vi "Main Page.vi"(8 "error in (no error)":errorcluster, 11 "Node Ptr":T3 format="%.0x") -> (0 "error out":errorcluster)   [LabVIEW 2023, in "Instrument Addon System Explorer.lvlib"]
uses:
  Instrument Addon System Explorer.lvlib
  <vilib>/NI VeriStand/Custom Device API/Custom Device Item Ref.ctl
  Addon Shared/Types/FG Control.ctl
  <vilib>/NI/NI VeriStand Hardware Resource Discovery/_Types/Filter Type.ctl
  Addon Shared/SubVIs/Constants.vi
  <vilib>/NI/NI VeriStand Advanced SysDef API/SysDef API/SysDef.Property.Get.vi
  <vilib>/NI/NI VeriStand Advanced SysDef API/_SubVIs/SysDef.Property.Get.String.vi
  <vilib>/NI/NI VeriStand Advanced SysDef API/SysDef API/SysDef.Property.Set.vi
  <vilib>/NI/NI VeriStand Advanced SysDef API/_SubVIs/SysDef.Property.Set.String.vi
  <vilib>/NI VeriStand/Custom Device API/NI VeriStand - Get Item Property.vi
  <vilib>/NI VeriStand/Custom Device API/Get Item Property (Boolean).vi
  <vilib>/NI VeriStand/Custom Device API/Get Item Property (U32).vi
  <vilib>/NI VeriStand/Custom Device API/Get Item Property (String).vi
  <vilib>/NI VeriStand/Custom Device API/NI VeriStand - Set Item Property.vi
  <vilib>/NI VeriStand/Custom Device API/Set Item Property (Boolean).vi
  <vilib>/NI VeriStand/Custom Device API/Set Item Property (U32).vi
  <vilib>/NI VeriStand/Custom Device API/Set Item Property (String).vi
  <vilib>/Utility/LVClass/Get LV Class Default Value.vi
  Includes/Protocols.lvlibp/Protocol Parent/Protocol Parent.lvclass
  <vilib>/NI VeriStand/Custom Device API/Custom Device API.lvlib
  Addon Shared/Instrument Addon Shared.lvlib
  <vilib>/NI/NI VeriStand Hardware Resource Discovery/NIVS Hardware Discovery.lvlib
  APIs/Scripting API/Instrument Addon Scripting API.lvlib
panel:
  out "Version":string
  in  "PCL Decimation":u32=1 min=1 max=10000 step=1
  in  "Protocol Settings":T1(tab)=enum."TCP/IP"
  in  "4wireMode":bool=TRUE caption="Specify Wire Mode"
  in  "COM Browse":bool
  in  "Termination Character":u8=10 format="%.0x"
  in  "End Write":bool=TRUE caption="End Write on Termination Character?"
  in  "End Read":bool=TRUE caption="End Read on Termination Character?"
  in  "XOFF":T2(ring)=enum."DC3"
  in  "XON":T2(ring)=enum."DC1"
  in  "Flow Control":u16(ring) items=["None"=0, "XON/XOFF"=1, "RTS/CTS"=2, "DTR/DSR"=4]
  in  "Stop Bits":u16(ring)=10 items=["1.0"=10, "1.5"=15, "2.0"=20]
  in  "Parity":enum16{"None", "Odd", "Even", "Mark", "Space"}(ring)
  in  "Data Bits":u16=8 min=5 max=8 step=1
  in  "Baud Rate":u32(ring)=9600 items=["75"=75, "110"=110, "134"=134, "150"=150, "300"=300, "600"=600, "1200"=1200, "1800"=1800, "2400"=2400, "4800"=4800, "7200"=7200, "9600"=9600, "14400"=14400, "19200"=19200, "28800"=28800, "38400"=38400, "56000"=56000, "57600"=57600, "115200"=115200, "128000"=128000, "230400"=230400, "460800"=460800, "921600"=921600, "1843200"=1843200, "3000000"=3000000]
  in  "Port":string="COM1"
  in  "WireMode":i16(ring)=-1 items=["Unknown"=-1, "RS485/Wire4"=0, "RS485/Wire2-EchoDTR"=1, "RS485/Wire2-CtrlDTR"=2, "RS485/Wire2-Auto"=3, "RS232/DTE"=128, "RS232/DCE"=129, "RS232/Auto"=130]
  in  "Assert DTR":bool=TRUE
  in  "VISA Browse":bool
  in  "Append Write Termination Character":bool caption="Append Write Termination Character?"
  in  "Timeout":u32=2000 caption="Timeout (ms)"
  in  "Termination Character":u8=10 format="%.0x"
  in  "Enable Termination Character":bool=TRUE caption="Enable Termination Character?"
  in  "VISA Resource":string="GPIB0::2::INSTR"
  in  "Port":u16
  in  "IP Address":string="localhost"
  in  "UDP Browse":bool
  in  "Target Port":u16
  in  "Target IP Address":string="localhost"
  in  "Local Port":u16
  in  "Local IP Address":string="localhost"
  in  "Assert REN w/ IFC":bool=TRUE caption="Assert REN w/ IFC?"
  in  "IST Bit Sense":bool=TRUE caption="IST Bit Sense?"
  in  "System Controller":bool=TRUE caption="System Controller?"
  in  "GPIB Address":string="1"
  in  "ConvBox Address":string="0"
  in  "ConvBox Browse":bool
  in  "ConvBox Port":string="COM1"
  in  "Protocol":string(combo)
  in  "SHDocVw.IWebBrowser":refnum<k7>(container)
  in  "Header":cluster{"Section Name":string}={"Section Name"="Addon Settings"}
  in  "Description":string
  in  "Name":string
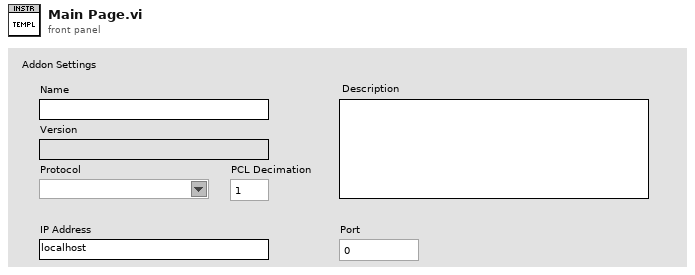
[diagram p1: front panel]
types:
  T1 = enum32{"RS232", "VISA", "TCP/IP", "UDP", "ConvBox"}
  T2 = enum16{"NUL", "SOH", "STX", "ETX", "EOT", "ENQ", "ACK", "BEL", "BS", "HT", "LF", "VT", "FF", "CR", "SO", "SI", "DLE", "DC1", "DC2", "DC3", "DC4", "NAK", "SYN", "ETB", "CAN", "EM", "SUB", "ESC", "FS", "GS", "RS", "US", "SP", "!", "\"", "#", "$", "%", "&", "'", "(", ")", "*", "+", ",", "- (-)", ".", "/", "0", "1", "2", "3", "4", "5", "6", "7", "8", "9", ":", ";", "<", "=", ">", "?", "@", "A", "B", "C", "D", "E", "F", "G", "H", "I", "J", "K", "L", "M", "N", "O", "P", "Q", "R", "S", "T", "U", "V", "W", "X", "Y", "Z", "[", "\\", "]", "^", "_", "`", "a", "b", "c", "d", "e", "f", "g", "h", "i", "j", "k", "l", "m", "n", "o", "p", "q", "r", "s", "t", "u", "v", "w", "x", "y", "z", "{", "|", "}", "~"}
  T3 = typedef "Custom Device API.lvlib/Custom Device Item Ref.ctl" = u64
  T4 = typedef "Instrument Addon Shared.lvlib/FG Control.ctl" = enum16{"Get", "Set"}
  T5 = typedef "NIVS Hardware Discovery.lvlib/Filter Type.ctl" = enum16{"Device Category", "Product Name", "Ethernet", "XNET", "VISA", "FPGA", "EtherCAT Master", "DAQmx", "GPIB", "Serial"}
  T6 = typedef "Custom Device API.lvlib/Custom Device Commands.ctl" = enum16{"Default", "Item renamed", "Shutdown", "Dynamic button pressed"}
  T7 = typedef "Instrument Addon Shared.lvlib/VISA Settings.ctl" = cluster{"VISA Resource":string, "Enable Termination Character":bool, "Termination Character":u8, "Timeout":u32, "Append Write Termination Character":bool}
  T8 = typedef "Instrument Addon Shared.lvlib/TCPIP Settings.ctl" = cluster{"IP Address":string, "Port":u16}
  T9 = typedef "Instrument Addon Shared.lvlib/UDP Settings.ctl" = cluster{"Local IP Address":string, "Local Port":u16, "Target IP Address":string, "Target Port":u16}
  T10 = typedef "Instrument Addon Shared.lvlib/RSXXX Port Settings.ctl" = cluster{"Port":string, "Baud Rate":u32, "Data Bits":u16, "Parity":enum16{"None", "Odd", "Even", "Mark", "Space"}, "Stop Bits":u16, "Flow Control":u16, "XON":enum16{"NUL", "SOH", "STX", "ETX", "EOT", "ENQ", "ACK", "BEL", "BS", "HT", "LF", "VT", "FF", "CR", "SO", "SI", "DLE", "DC1", "DC2", "DC3", "DC4", "NAK", "SYN", "ETB", "CAN", "EM", "SUB", "ESC", "FS", "GS", "RS", "US", "SP", "!", "\"", "#", "$", "%", "&", "'", "(", ")", "*", "+", ",", "- (-)", ".", "/", "0", "1", "2", "3", "4", "5", "6", "7", "8", "9", ":", ";", "<", "=", ">", "?", "@", "A", "B", "C", "D", "E", "F", "G", "H", "I", "J", "K", "L", "M", "N", "O", "P", "Q", "R", "S", "T", "U", "V", "W", "X", "Y", "Z", "[", "\\", "]", "^", "_", "`", "a", "b", "c", "d", "e", "f", "g", "h", "i", "j", "k", "l", "m", "n", "o", "p", "q", "r", "s", "t", "u", "v", "w", "x", "y", "z", "{", "|", "}", "~"}, "XOFF":enum16{"NUL", "SOH", "STX", "ETX", "EOT", "ENQ", "ACK", "BEL", "BS", "HT", "LF", "VT", "FF", "CR", "SO", "SI", "DLE", "DC1", "DC2", "DC3", "DC4", "NAK", "SYN", "ETB", "CAN", "EM", "SUB", "ESC", "FS", "GS", "RS", "US", "SP", "!", "\"", "#", "$", "%", "&", "'", "(", ")", "*", "+", ",", "- (-)", ".", "/", "0", "1", "2", "3", "4", "5", "6", "7", "8", "9", ":", ";", "<", "=", ">", "?", "@", "A", "B", "C", "D", "E", "F", "G", "H", "I", "J", "K", "L", "M", "N", "O", "P", "Q", "R", "S", "T", "U", "V", "W", "X", "Y", "Z", "[", "\\", "]", "^", "_", "`", "a", "b", "c", "d", "e", "f", "g", "h", "i", "j", "k", "l", "m", "n", "o", "p", "q", "r", "s", "t", "u", "v", "w", "x", "y", "z", "{", "|", "}", "~"}, "End Read on Termination Character":bool, "End Write on Termination Character":bool, "Termination Character":u8, "4wireMode":bool, "AssertDTR":bool, "WireMode":i16}
  T11 = typedef "Instrument Addon Shared.lvlib/GPIB ConvBox Settings.ctl" = cluster{"Port":string, "ConvBox Address":string, "Assert Ren with IFC":bool, "System controller":bool, "IST bit sense":bool, "GPIB Address":string}
  T12 = typedef "Protocols.lvlibp/Protocol Parent.lvclass/Base Protocol Type.ctl" = enum16{"RS-XXX", "VISA", "TCPIP", "UDP", "GPIB ConvBox"}
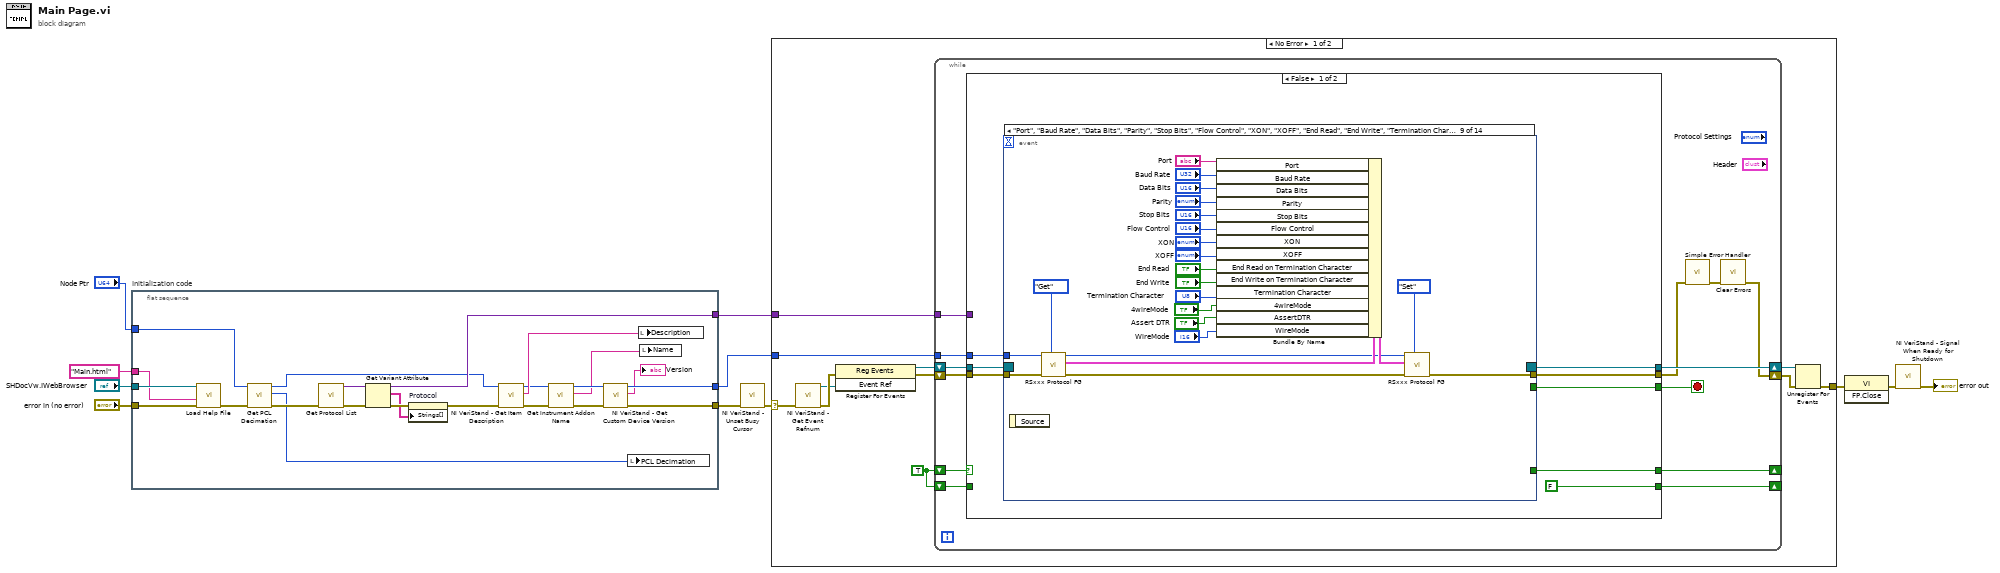
[diagram p0: block diagram]
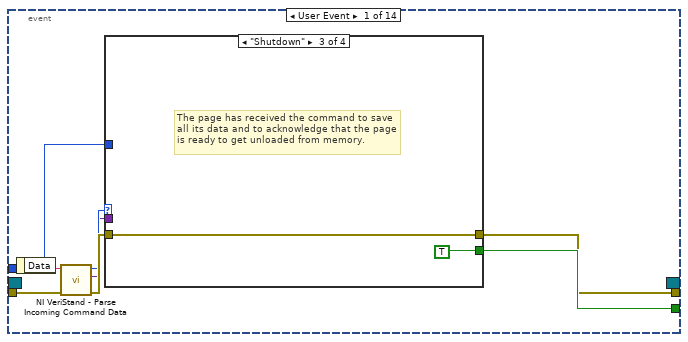
[diagram p2: hidden frame]
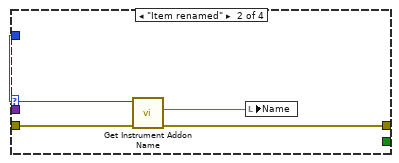
[diagram p4: hidden frame]
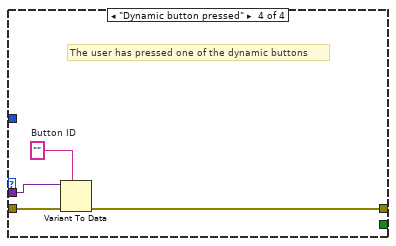
[diagram p5: hidden frame]
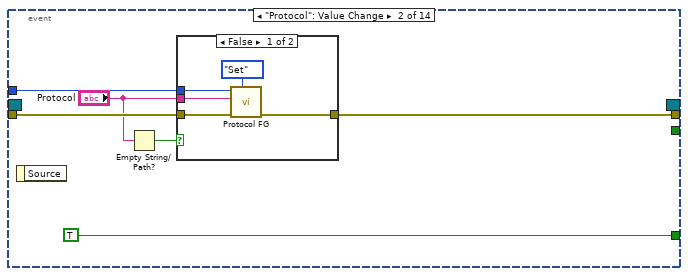
[diagram p6: hidden frame]
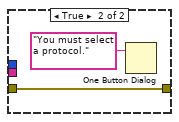
[diagram p7: hidden frame]
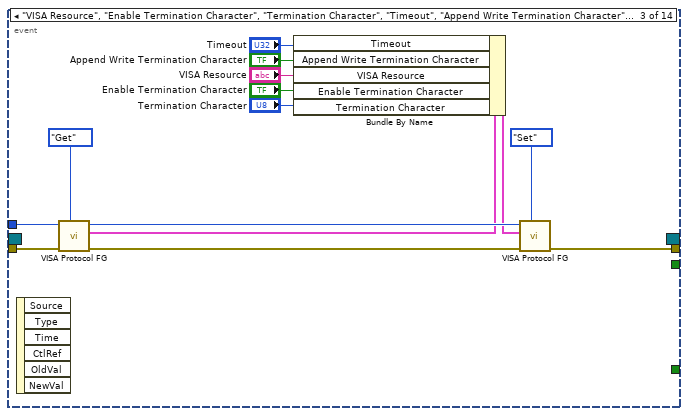
[diagram p8: hidden frame]
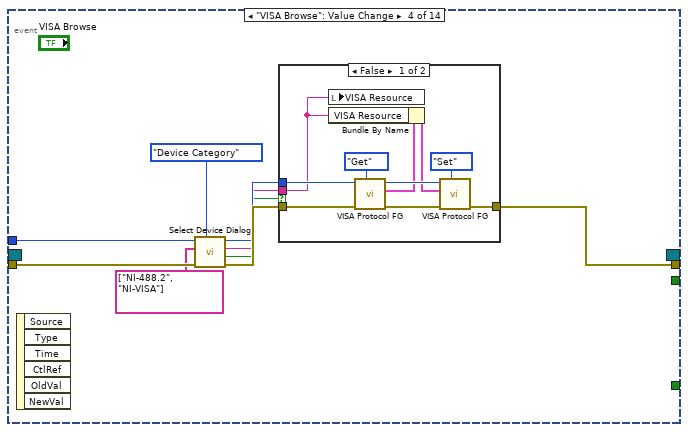
[diagram p9: hidden frame]
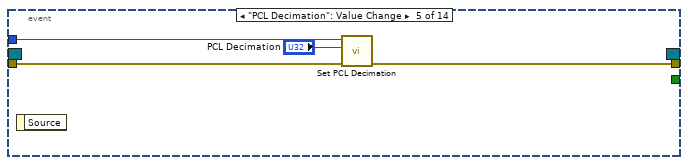
[diagram p11: hidden frame]
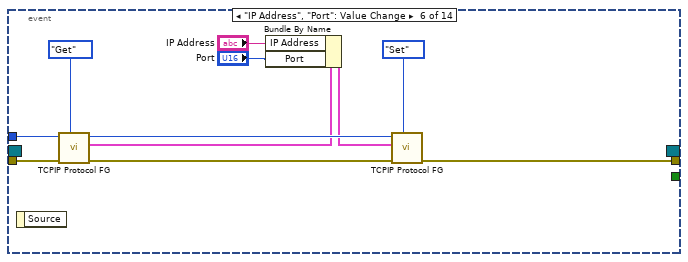
[diagram p12: hidden frame]
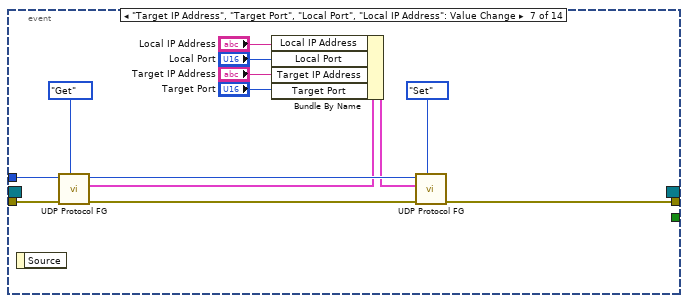
[diagram p13: hidden frame]
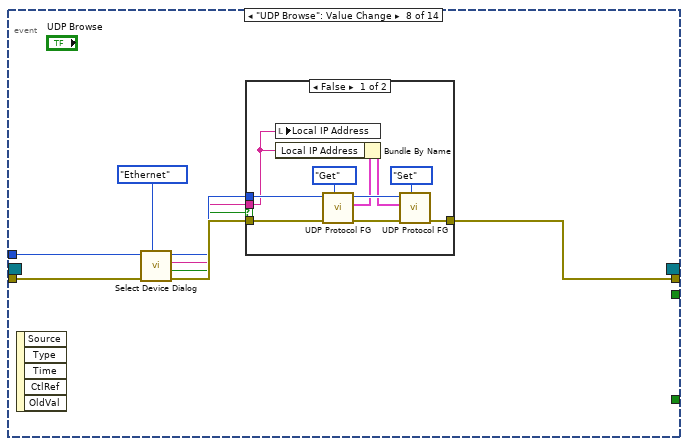
[diagram p14: hidden frame]
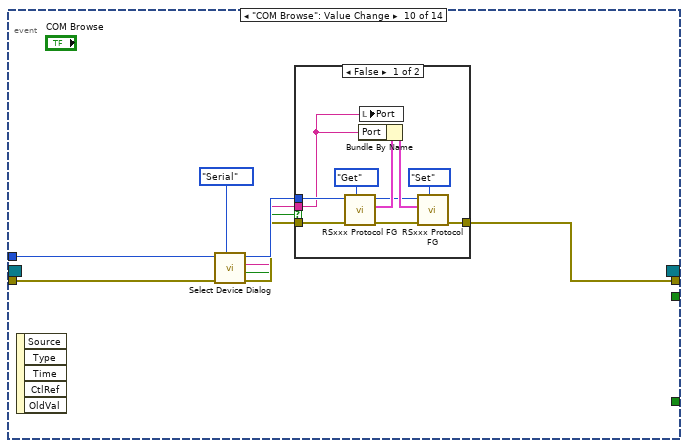
[diagram p16: hidden frame]
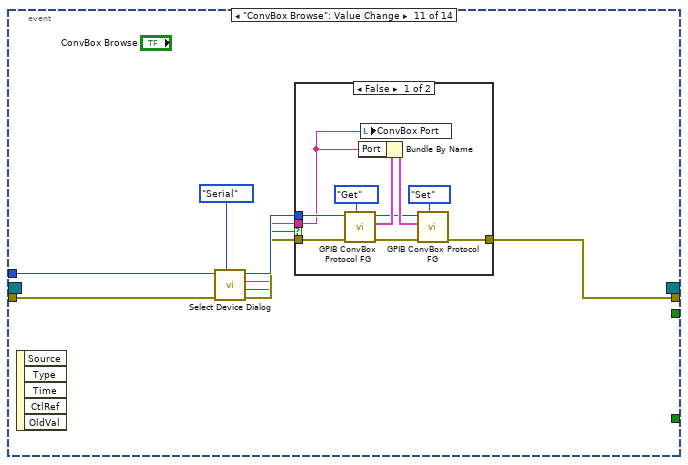
[diagram p18: hidden frame]
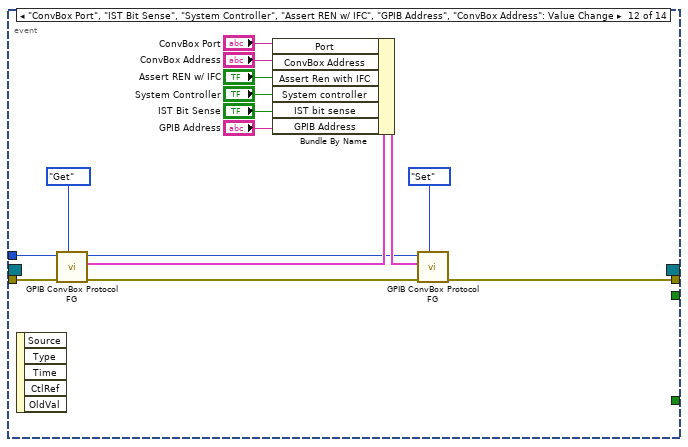
[diagram p20: hidden frame]
diagram:
  n1 = flat-sequence "Initialization code" {
    tunnel: "error in (no error)" -> [w33]
    tunnel: "Node Ptr" -> [w19]
    tunnel: [w24] -> w7
    tunnel: [w23] -> w4
    tunnel: "SHDocVw.IWebBrowser" -> [w32]
    tunnel: "Main.html" ("HTML File") -> [w31]
    tunnel: [w26] -> w1
    frame #0 {
      n2 = call "Load Help File.vi"("error in (no error)"=w33, "HTML File to Load"=w31, "SHDocVw.IWebBrowser2"=w32) -> ("error out"=w21:errorcluster)  [unwired: 8 in]
      n3 = call "Get PCL Decimation.vi"("error in (no error)"=w21, "instrument addon refnum in"=w19) -> ("error out"=w20:errorcluster, "PCL decimation"=w17:u32, "instrument addon refnum out"=w18:T3)  [unwired: 7 in]
      n4 = call "Get Protocol List.vi"("error in (no error)"=w20) -> ("error out"=w29:errorcluster, "Class Lookup"=w30:variant)  [unwired: 9 in]
      n5 = Get Variant Attribute(Variant=w30, error in=w29) -> (duplicate Variant=w26:variant, names=w27:string[], error out=w28:errorcluster)  [unwired: 2 in, 1 out]
      n6 = property on="Protocol" class="CmbBox"(error in=w28, "Strings[]"=w27) -> (error out=w25:errorcluster)  [unwired: 1 in, 1 out]
      n7 = call <vilib>:"NI VeriStand - Get Item Description.vi"("error in (no error)"=w25, "Item Ref in"=w18) -> ("error out"=w16:errorcluster, "Description"=w34:string, "Item Ref out"=w14:T3)  [unwired: 7 out]
      n8 = call "Get Instrument Addon Name.vi"("error in (no error)"=w16, "instrument addon refnum in"=w14) -> ("error out"=w15:errorcluster, "name"=w12:string, "instrument addon refnum out"=w13:T3)  [unwired: 7 in]
      n9 = call <vilib>:"NI VeriStand - Get Custom Device Version.vi"("error in (no error)"=w15, "Device Ref in"=w13) -> ("error out"=w24:errorcluster, "Value"=→"Version":string, "Device Ref out"=w23:T3)  [unwired: 7 in]
      n10 = local write "PCL Decimation"(w17) -> ()
      n11 = local write "Description"(w34) -> ()
      n12 = local write "Name"(w12) -> ()
    }
  }
  n13 = call <vilib>:"NI VeriStand - Unset Busy Cursor.vi"("error in (no error)"=w7) -> ("error out"=w6:errorcluster)  [unwired: 10 out]
  n14 = case shown="No Error" w6 {
    selector: w6 -> [w37 w349]
    tunnel: [w42 w347] -> w11
    tunnel: w4 -> [w38 _]
    tunnel: w1 -> [w36 _]
    frame No Error {
      w35 = TRUE
      n15 = call <vilib>:"NI VeriStand - Get Event Refnum.vi"("error in (no error)"=w37) -> ("error out"=w45:errorcluster, "Event Ref"=w41:refnum<user-event>)  [unwired: 9 out]
      n16 = register-events(error in=w45, w41) -> (reference out=w39:refnum<event-registration>, error out=w40:errorcluster)  [unwired: 1 in]
      n17 = while {
        tunnel: w38 -> [w54]
        shift-right: [w51] -> w43
        shift-left: w40 -> [w57]
        shift-right: [w58] -> w44
        shift-left: w39 -> [w56]
        tunnel: w36 -> [w50]
        shift-right: [w48] -> _
        shift-left: w35 -> [w49]
        shift-right: [w46] -> _
        shift-left: w35 -> [w47]
        stop <- w55 stop-if-true
        n18 = case shown="False" w49 {
          tunnel: [w66 w271] -> w58
          tunnel: w57 -> [w65 w279]
          tunnel: w56 -> [w64 w271]
          tunnel: [w63 _] -> w55
          tunnel: w54 -> [w62 w278]
          tunnel: [w61 w266] -> w53
          tunnel: w50 -> [_ w276]
          tunnel: [w60 w264] -> w48
          tunnel: w47 -> [_ w265]
          tunnel: [FALSE w264] -> w46
          frame False {
            n19 = event shown="[8] \"Port\", \"Baud Rate\", \"Data Bits\", \"Parity\", \"Stop Bits\", \"Flow Control\", \"XON\", \"XOFF\", \"End Read\", \"End Write\", \"Termination Character\", \"4wireMode\", \"Assert DTR\", \"WireMode\": Value Change" {
              selector: w64 -> [_ _ _ _ _ _ _ _ _ _ _ _ _ _]
              dyn-events: [_ _ _ _ _ _ _ _ _ _ _ _ _ _] -> w66
              timeout: _ -> [_ _ _ _ _ _ _ _ _ _ _ _ _ _]
              tunnel: w65 -> [w74 w90 w111 w120 w136 w146 w159 w167 w199 w209 w228 w248 w259 w262]
              tunnel: [w70 _ _ _ _ _ _ _ _ _ _ _ _ _] -> w63
              tunnel: [w69 w86 w107 w121 w135 w142 w155 w168 w201 w210 w229 w255 w258 w261] -> w61
              tunnel: w62 -> [w68 w91 w110 w118 w133 w145 w158 w165 w197 w208 w227 w247 w256 w263]
              tunnel: [_ TRUE _ _ _ _ _ _ _ _ _ _ _ _] -> w60
              event User Event {
                n20 = event-data() -> ("Data"=w73:string)  [unwired: 1 out]
                n21 = call <vilib>:"NI VeriStand - Parse Incoming Command Data.vi"("error in (no error)"=w74, "Incoming data"=w73) -> ("error out"=w72:errorcluster, "Outgoing data"=w67:variant, "Action"=w71:T6)  [unwired: 7 out]
                n22 = case shown="\"Shutdown\"" w71 {
                  tunnel: w72 -> [w75 w77 w80 w85]
                  tunnel: [_ _ TRUE _] -> w70
                  tunnel: [w75 w76 w80 w82] -> w69
                  tunnel: w68 -> [_ w78 _ _]
                  tunnel: w67 -> [_ _ _ w84]
                  frame "Default", Default {
                  }
                  frame "Item renamed" {
                    n23 = call "Get Instrument Addon Name.vi"("error in (no error)"=w77, "instrument addon refnum in"=w78) -> ("error out"=w76:errorcluster, "name"=w79:string)  [unwired: 7 in, 1 out]
                    n24 = local write "Name"(w79) -> ()
                  }
                  frame "Shutdown" {
                    # "The page has received the command to save all its data and to acknowledge that the page is ready to get unloaded from memory."
                  }
                  frame "Dynamic button pressed" {
                    w83 = ""  # Button ID
                    # "The user has pressed one of the dynamic buttons"
                    n25 = Variant To Data(error in=w85, type=w83, Variant=w84) -> (error out=w82:errorcluster)  [unwired: 1 out]
                  }
                }
              }
              event "Protocol": Value Change {
                n26 = event-data() -> ()  [unwired: 2 out]
                n27 = Empty String/Path?(string/path="Protocol") -> (empty?=w88:bool)
                n28 = case shown="False" w88 {
                  tunnel: w91 -> [w94 _]
                  tunnel: w90 -> [w95 w97]
                  tunnel: [w92 w97] -> w86
                  tunnel: "Protocol" -> [w93 _]
                  frame False {
                    n29 = call "Protocol FG.vi"("Action"=FG_Control."Set", "error in (no error)"=w95, "Protocol"=w93, "Device Item Ref in"=w94) -> ("error out"=w92:errorcluster)  [unwired: 5 in, 2 out]
                  }
                  frame True {
                    n30 = One Button Dialog(message="You must select a protocol.") -> ()  [unwired: 1 in, 1 out]
                  }
                }
              }
              event "VISA Resource", "Enable Termination Character", "Termination Character", "Timeout", "Append Write Termination Character": Value Change {
                n31 = event-data() -> ()  [unwired: 7 out]
                n32 = call "VISA Protocol FG.vi"("Action"=FG_Control."Get", "error in (no error)"=w111, "Device Item Ref in"=w110) -> ("error out"=w108:errorcluster, "VISA Config"=w105:T7, "Item Ref out"=w106:T3)  [unwired: 6 in]
                n33 = Bundle By Name(cluster=w105, "Timeout"="Timeout", "Append Write Termination Character"="Append Write Termination Character", "VISA Resource"="VISA Resource", "Enable Termination Character"="Enable Termination Character", "Termination Character"="Termination Character") -> (w104:T7)
                n34 = call "VISA Protocol FG.vi"("Action"=FG_Control."Set", "error in (no error)"=w108, "VISA Config"=w104, "Device Item Ref in"=w106) -> ("error out"=w107:errorcluster)  [unwired: 5 in, 2 out]
              }
              event "VISA Browse": Value Change {
                n35 = event-data() -> ()  [unwired: 7 out]
                n36 = call <vilib>:"Select Device Dialog.vi"("Filter Type"=Filter_Type."Device Category", "error in (no error)"=w120, "Filter Names"=string[] ["NI-488.2", "NI-VISA"], "Item Ref in"=w118) -> ("error out"=w119:errorcluster, "Cancelled?"=w116:bool, "Selected Alias"=w115:string, "Item Ref out"=w117:T3)  [unwired: 4 in]
                n37 = case shown="False" w116 {
                  tunnel: w119 -> [w130 w132]
                  tunnel: w117 -> [w129 _]
                  tunnel: [w126 w132] -> w121
                  tunnel: w115 -> [w122 _]
                  frame False {
                    n38 = local write "VISA Resource"(w122) -> ()
                    n39 = call "VISA Protocol FG.vi"("Action"=FG_Control."Get", "error in (no error)"=w130, "Device Item Ref in"=w129) -> ("error out"=w127:errorcluster, "VISA Config"=w124:T7, "Item Ref out"=w125:T3)  [unwired: 6 in]
                    n40 = Bundle By Name(cluster=w124, "VISA Resource"=w122) -> (w123:T7)
                    n41 = call "VISA Protocol FG.vi"("Action"=FG_Control."Set", "error in (no error)"=w127, "VISA Config"=w123, "Device Item Ref in"=w125) -> ("error out"=w126:errorcluster)  [unwired: 5 in, 2 out]
                  }
                  frame True {
                  }
                }
              }
              event "PCL Decimation": Value Change {
                n42 = event-data() -> ()  [unwired: 2 out]
                n43 = call "Set PCL Decimation.vi"("error in (no error)"=w136, "PCL decimation"="PCL Decimation", "instrument addon refnum in"=w133) -> ("error out"=w135:errorcluster)  [unwired: 7 in, 1 out]
              }
              event "IP Address", "Port": Value Change {
                n44 = event-data() -> ()  [unwired: 2 out]
                n45 = call "TCPIP Protocol FG.vi"("Action"=FG_Control."Get", "error in (no error)"=w146, "Device Item Ref in"=w145) -> ("error out"=w143:errorcluster, "TCP/IP Config"=w140:T8, "Item Ref out"=w141:T3)  [unwired: 6 in]
                n46 = Bundle By Name(cluster=w140, "IP Address"="IP Address", "Port"="Port") -> (w139:T8)
                n47 = call "TCPIP Protocol FG.vi"("Action"=FG_Control."Set", "error in (no error)"=w143, "TCP/IP Config"=w139, "Device Item Ref in"=w141) -> ("error out"=w142:errorcluster)  [unwired: 5 in, 2 out]
              }
              event "Target IP Address", "Target Port", "Local Port", "Local IP Address": Value Change {
                n48 = event-data() -> ()  [unwired: 2 out]
                n49 = call "UDP Protocol FG.vi"("Action"=FG_Control."Get", "error in (no error)"=w159, "Device Item Ref in"=w158) -> ("error out"=w156:errorcluster, "UDP Config"=w153:T9, "Item Ref out"=w154:T3)  [unwired: 6 in]
                n50 = Bundle By Name(cluster=w153, "Local IP Address"="Local IP Address", "Local Port"="Local Port", "Target IP Address"="Target IP Address", "Target Port"="Target Port") -> (w152:T9)
                n51 = call "UDP Protocol FG.vi"("Action"=FG_Control."Set", "error in (no error)"=w156, "UDP Config"=w152, "Device Item Ref in"=w154) -> ("error out"=w155:errorcluster)  [unwired: 5 in, 2 out]
              }
              event "UDP Browse": Value Change {
                n52 = event-data() -> ()  [unwired: 6 out]
                n53 = call <vilib>:"Select Device Dialog.vi"("Filter Type"=Filter_Type."Ethernet", "error in (no error)"=w167, "Item Ref in"=w165) -> ("error out"=w166:errorcluster, "Cancelled?"=w163:bool, "Selected Alias"=w162:string, "Item Ref out"=w164:T3)  [unwired: 5 in]
                n54 = case shown="False" w163 {
                  tunnel: w166 -> [w177 w179]
                  tunnel: w164 -> [w176 _]
                  tunnel: [w173 w179] -> w168
                  tunnel: w162 -> [w169 _]
                  frame False {
                    n55 = local write "Local IP Address"(w169) -> ()
                    n56 = call "UDP Protocol FG.vi"("Action"=FG_Control."Get", "error in (no error)"=w177, "Device Item Ref in"=w176) -> ("error out"=w174:errorcluster, "UDP Config"=w171:T9, "Item Ref out"=w172:T3)  [unwired: 6 in]
                    n57 = Bundle By Name(cluster=w171, "Local IP Address"=w169) -> (w170:T9)
                    n58 = call "UDP Protocol FG.vi"("Action"=FG_Control."Set", "error in (no error)"=w174, "UDP Config"=w170, "Device Item Ref in"=w172) -> ("error out"=w173:errorcluster)  [unwired: 5 in, 2 out]
                  }
                  frame True {
                  }
                }
              }
              event "Port", "Baud Rate", "Data Bits", "Parity", "Stop Bits", "Flow Control", "XON", "XOFF", "End Read", "End Write", "Termination Character", "4wireMode", "Assert DTR", "WireMode": Value Change {
                n59 = event-data() -> ()  [unwired: 2 out]
                n60 = call "RSxxx Protocol FG.vi"("Action"=FG_Control."Get", "error in (no error)"=w199, "Device Item Ref in"=w197) -> ("error out"=w198:errorcluster, "Serial Config"=w196:T10, "Item Ref out"=w183:T3)  [unwired: 6 in]
                n61 = Bundle By Name(cluster=w196, "Port"="Port", "Baud Rate"="Baud Rate", "Data Bits"="Data Bits", "Parity"="Parity", "Stop Bits"="Stop Bits", "Flow Control"="Flow Control", "XON"="XON", "XOFF"="XOFF", "End Read on Termination Character"="End Read", "End Write on Termination Character"="End Write", "Termination Character"="Termination Character", "4wireMode"="4wireMode", "AssertDTR"="Assert DTR", "WireMode"="WireMode") -> (w195:T10)
                n62 = call "RSxxx Protocol FG.vi"("Action"=FG_Control."Set", "error in (no error)"=w198, "Serial Config"=w195, "Device Item Ref in"=w183) -> ("error out"=w201:errorcluster)  [unwired: 5 in, 2 out]
              }
              event "COM Browse": Value Change {
                n63 = event-data() -> ()  [unwired: 6 out]
                n64 = call <vilib>:"Select Device Dialog.vi"("Filter Type"=Filter_Type."Serial", "error in (no error)"=w209, "Item Ref in"=w208) -> ("error out"=w206:errorcluster, "Cancelled?"=w205:bool, "Selected Alias"=w204:string, "Item Ref out"=w207:T3)  [unwired: 5 in]
                n65 = case shown="False" w205 {
                  tunnel: [w219 w221] -> w210
                  tunnel: w206 -> [w217 w221]
                  tunnel: w207 -> [w215 _]
                  tunnel: w204 -> [w211 _]
                  frame False {
                    n66 = call "RSxxx Protocol FG.vi"("Action"=FG_Control."Get", "error in (no error)"=w217, "Device Item Ref in"=w215) -> ("error out"=w216:errorcluster, "Serial Config"=w214:T10, "Item Ref out"=w212:T3)  [unwired: 6 in]
                    n67 = Bundle By Name(cluster=w214, "Port"=w211) -> (w213:T10)
                    n68 = local write "Port"(w211) -> ()
                    n69 = call "RSxxx Protocol FG.vi"("Action"=FG_Control."Set", "error in (no error)"=w216, "Serial Config"=w213, "Device Item Ref in"=w212) -> ("error out"=w219:errorcluster)  [unwired: 5 in, 2 out]
                  }
                  frame True {
                  }
                }
              }
              event "ConvBox Browse": Value Change {
                n70 = event-data() -> ()  [unwired: 6 out]
                n71 = call <vilib>:"Select Device Dialog.vi"("Filter Type"=Filter_Type."Serial", "error in (no error)"=w228, "Item Ref in"=w227) -> ("error out"=w225:errorcluster, "Cancelled?"=w224:bool, "Selected Alias"=w223:string, "Item Ref out"=w226:T3)  [unwired: 5 in]
                n72 = case shown="False" w224 {
                  tunnel: [w238 w240] -> w229
                  tunnel: w225 -> [w236 w240]
                  tunnel: w226 -> [w234 _]
                  tunnel: w223 -> [w230 _]
                  frame False {
                    n73 = call "GPIB ConvBox Protocol FG.vi"("Action"=FG_Control."Get", "error in (no error)"=w236, "Device Item Ref in"=w234) -> ("error out"=w235:errorcluster, "GPIB ConvBox Config"=w233:T11, "Item Ref out"=w231:T3)  [unwired: 6 in]
                    n74 = Bundle By Name(cluster=w233, "Port"=w230) -> (w232:T11)
                    n75 = local write "ConvBox Port"(w230) -> ()
                    n76 = call "GPIB ConvBox Protocol FG.vi"("Action"=FG_Control."Set", "error in (no error)"=w235, "GPIB ConvBox Config"=w232, "Device Item Ref in"=w231) -> ("error out"=w238:errorcluster)  [unwired: 5 in, 2 out]
                  }
                  frame True {
                  }
                }
              }
              event "ConvBox Port", "IST Bit Sense", "System Controller", "Assert REN w/ IFC", "GPIB Address", "ConvBox Address": Value Change {
                n77 = event-data() -> ()  [unwired: 6 out]
                n78 = call "GPIB ConvBox Protocol FG.vi"("Action"=FG_Control."Get", "error in (no error)"=w248, "Device Item Ref in"=w247) -> ("error out"=w252:errorcluster, "GPIB ConvBox Config"=w251:T11, "Item Ref out"=w249:T3)  [unwired: 6 in]
                n79 = Bundle By Name(cluster=w251, "Port"="ConvBox Port", "ConvBox Address"="ConvBox Address", "Assert Ren with IFC"="Assert REN w/ IFC", "System controller"="System Controller", "IST bit sense"="IST Bit Sense", "GPIB Address"="GPIB Address") -> (w250:T11)
                n80 = call "GPIB ConvBox Protocol FG.vi"("Action"=FG_Control."Set", "error in (no error)"=w252, "GPIB ConvBox Config"=w250, "Device Item Ref in"=w249) -> ("error out"=w255:errorcluster)  [unwired: 5 in, 2 out]
              }
              event "Name": Value Change {
                n81 = event-data() -> ()  [unwired: 2 out]
                n82 = call "Set Instrument Addon Name.vi"("error in (no error)"=w259, "name"="Name", "instrument addon refnum in"=w256) -> ("error out"=w258:errorcluster)  [unwired: 7 in, 1 out]
              }
              event "Description": Value Change {
                n83 = event-data() -> ()  [unwired: 2 out]
                n84 = call <vilib>:"NI VeriStand - Set Item Description.vi"("error in (no error)"=w262, "Description"="Description", "Item Ref in"=w263) -> ("error out"=w261:errorcluster)  [unwired: 8 out]
              }
            }
          }
          frame True {
            w264 = FALSE
            n85 = call "Protocol FG.vi"("Action"=FG_Control."Get", "error in (no error)"=w279, "Device Item Ref in"=w278) -> ("error out"=w275:errorcluster, "Protocol out"=w272:string, "Item Ref out"=w274:T3)  [unwired: 6 in]
            n86 = call "Lookup Base Protocol Class and Info.vi"("error in (no error)"=w275, "Protocol in"=w272, "Class Lookup"=w276) -> ("error out"=w277:errorcluster, "Protocol out"=w270:T12, "Error Codes"=w269:cluster{"Code":i32, "String":string}[])  [unwired: 4 in, 2 out]
            n87 = case shown="\"RS-XXX\"" w270 {
              tunnel: w277 -> [w296 w304 w314 w334 w346]
              tunnel: [w295 w303 w313 w333 w345] -> w267
              tunnel: w274 -> [w294 w302 w312 w332 w344]
              tunnel: [w286 w297 w305 w318 w335] -> w268
              frame "VISA" {
                n88 = call "VISA Protocol FG.vi"("Action"=FG_Control."Get", "error in (no error)"=w296, "Device Item Ref in"=w294) -> ("error out"=w295:errorcluster, "VISA Config"=w292:T7, "Item Ref out"=w286:T3)  [unwired: 6 in]
                n89 = Unbundle By Name(w292) -> ("Append Write Termination Character"=w287:bool, "Timeout"=w288:u32, "VISA Resource"=w291:string, "Enable Termination Character"=w290:bool, "Termination Character"=w289:u8)
                n90 = local write "Append Write Termination Character"(w287) -> ()
                n91 = local write "Enable Termination Character"(w290) -> ()
                n92 = local write "Termination Character"(w289) -> ()
                n93 = local write "Timeout"(w288) -> ()
                n94 = local write "VISA Resource"(w291) -> ()
              }
              frame "TCPIP" {
                n95 = call "TCPIP Protocol FG.vi"("Action"=FG_Control."Get", "error in (no error)"=w304, "Device Item Ref in"=w302) -> ("error out"=w303:errorcluster, "TCP/IP Config"=w300:T8, "Item Ref out"=w297:T3)  [unwired: 6 in]
                n96 = Unbundle By Name(w300) -> ("IP Address"=w299:string, "Port"=w298:u16)
                n97 = local write "IP Address"(w299) -> ()
                n98 = local write "Port"(w298) -> ()
              }
              frame "UDP" {
                n99 = call "UDP Protocol FG.vi"("Action"=FG_Control."Get", "error in (no error)"=w314, "Device Item Ref in"=w312) -> ("error out"=w313:errorcluster, "UDP Config"=w310:T9, "Item Ref out"=w305:T3)  [unwired: 6 in]
                n100 = Unbundle By Name(w310) -> ("Local IP Address"=w309:string, "Local Port"=w308:u16, "Target IP Address"=w307:string, "Target Port"=w306:u16)
                n101 = local write "Local IP Address"(w309) -> ()
                n102 = local write "Local Port"(w308) -> ()
                n103 = local write "Target IP Address"(w307) -> ()
                n104 = local write "Target Port"(w306) -> ()
              }
              frame "RS-XXX" {
                n105 = call "RSxxx Protocol FG.vi"("Action"=FG_Control."Get", "error in (no error)"=w334, "Device Item Ref in"=w332) -> ("error out"=w333:errorcluster, "Serial Config"=w330:T10, "Item Ref out"=w318:T3)  [unwired: 6 in]
                n106 = Unbundle By Name(w330) -> ("Port"=w329:string, "Baud Rate"=w328:u32, "Data Bits"=w319:u16, "Parity"=w320:enum16{"None", "Odd", "Even", "Mark", "Space"}, "Stop Bits"=w321:u16, "Flow Control"=w322:u16, "XON"=w323:T2, "XOFF"=w324:T2, "End Read on Termination Character"=w325:bool, "End Write on Termination Character"=w326:bool, "Termination Character"=w327:u8, "4wireMode"=w317:bool, "AssertDTR"=w316:bool, "WireMode"=w315:i16)
                n107 = local write "4wireMode"(w317) -> ()
                n108 = local write "Assert DTR"(w316) -> ()
                n109 = local write "Termination Character"(w327) -> ()
                n110 = local write "Flow Control"(w322) -> ()
                n111 = local write "End Write"(w326) -> ()
                n112 = local write "Baud Rate"(w328) -> ()
                n113 = local write "Data Bits"(w319) -> ()
                n114 = local write "Stop Bits"(w321) -> ()
                n115 = local write "XON"(w323) -> ()
                n116 = local write "End Read"(w325) -> ()
                n117 = local write "Port"(w329) -> ()
                n118 = local write "Parity"(w320) -> ()
                n119 = local write "XOFF"(w324) -> ()
                n120 = local write "WireMode"(w315) -> ()
              }
              frame "GPIB ConvBox" {
                n121 = call "GPIB ConvBox Protocol FG.vi"("Action"=FG_Control."Get", "error in (no error)"=w346, "Device Item Ref in"=w344) -> ("error out"=w345:errorcluster, "GPIB ConvBox Config"=w342:T11, "Item Ref out"=w335:T3)  [unwired: 6 in]
                n122 = Unbundle By Name(w342) -> ("Port"=w341:string, "ConvBox Address"=w340:string, "Assert Ren with IFC"=w339:bool, "System controller"=w338:bool, "IST bit sense"=w337:bool, "GPIB Address"=w336:string)
                n123 = local write "Assert REN w/ IFC"(w339) -> ()
                n124 = local write "IST Bit Sense"(w337) -> ()
                n125 = local write "ConvBox Port"(w341) -> ()
                n126 = local write "ConvBox Address"(w340) -> ()
                n127 = local write "System Controller"(w338) -> ()
                n128 = local write "GPIB Address"(w336) -> ()
              }
            }
            n129 = To Unsigned Long Integer(number=w270) -> (unsigned 32bit integer=w273:u32)
            n130 = local write "Protocol Settings"(w273) -> ()
            n131 = local write "Protocol"(w272) -> ()
            n132 = case shown="True" w265 {
              tunnel: w269 -> [w284 _]
              tunnel: w268 -> [w283 _]
              tunnel: w267 -> [w282 w285]
              tunnel: [w281 w285] -> w266
              frame False {
                n133 = call "Set Codes on all Error Channels.vi"("error in (no error)"=w282, "Error Codes"=w284, "Node Ptr in"=w283) -> ("error out"=w281:errorcluster)  [unwired: 7 in, 1 out]
              }
              frame True {
              }
            }
          }
        }
        n134 = call <vilib>:"Simple Error Handler.vi"("error in (no error)"=w53) -> ("error out"=w52:errorcluster)  [unwired: 1 in, 7 out]
        n135 = call <vilib>:"Clear Errors.vi"("error in (no error)"=w52) -> ("error out"=w51:errorcluster)  [unwired: 1 in, 5 out]
      }
      n136 = Unregister For Events(event registration refnum=w44, error in=w43) -> (error out=w42:errorcluster)
    }
    frame Error {
      n137 = call <vilib>:"Simple Error Handler.vi"("error in (no error)"=w349) -> ("error out"=w348:errorcluster)  [unwired: 1 in, 7 out]
      n138 = call <vilib>:"Clear Errors.vi"("error in (no error)"=w348) -> ("error out"=w347:errorcluster)  [unwired: 1 in, 5 out]
    }
  }
  n139 = invoke class="VI" method="FP.Close"(error in=w11) -> (error out=w10:errorcluster)  [unwired: 2 in, 2 out]
  n140 = call <vilib>:"NI VeriStand - Signal When Ready for Shutdown.vi"("error in (no error)"=w10) -> ("error out"=→"error out":errorcluster)  [unwired: 10 out]
